vi "Begin.vi"(8 "error in":errorcluster) -> (0 "error out":errorcluster)   [LabVIEW 2019]
doc: "Called before other user functions, this VI is expected to open initial I/O refnums, load in file data, and do all program initialization. Notice that the <B>error out</B> terminal is simply used for data flow. Wiring it to other structures or subVIs ensures that this VI runs first."
uses:
  <vilib>/Rock Robotics/WPI/Camera/WPI_CameraImageSize.ctl
  <vilib>/Rock Robotics/WPI/Camera/WPI_CameraFrameRate.ctl
  <vilib>/Rock Robotics/WPI/Camera/WPI_CameraWhite Balance Values.ctl
  <vilib>/Rock Robotics/WPI/Camera/WPI_CameraExposure Values.ctl
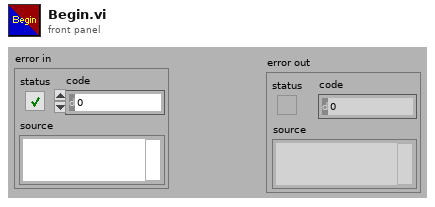
[diagram p1: front panel]
types:
  T1 = typedef "WPI_CameraExposure Values.ctl" = enum16{"Auto", "Flicker-free 50 Hz", "Flicker-free 60 Hz", "Hold current", "Custom"}
  T2 = typedef "WPI_CameraWhite Balance Values.ctl" = enum16{"Auto", "Fixed indoor", "Fixed outdoor 1", "Fixed outdoor 2", "Fixed fluorescent 1", "Fixed fluorescent 2", "Hold current", "Custom"}
  T3 = typedef "WPI_CameraFrameRate.ctl" = u32
  T4 = typedef "WPI_CameraImageSize.ctl" = enum16{"640x480", "320x240", "160x120", "Custom"}
  T5 = typedef "WPI_CameraDevRef.ctl" = cluster{"Camera Address":string, "CameraStatus":errorcluster}
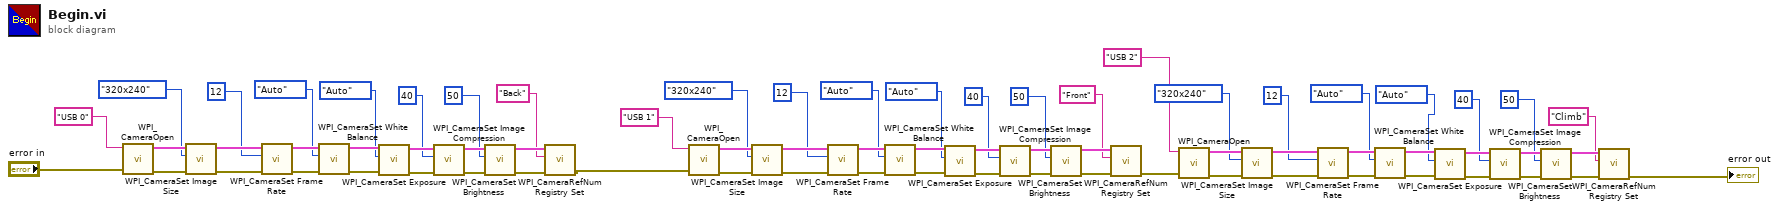
[diagram p0: block diagram]
diagram:
  n1 = call <vilib>:"WPI_CameraOpen.vi"("error in (no error)"="error in", "Camera Address"="USB 0") -> ("error out"=w68:errorcluster, "CameraDevRef"=w67:T5)  [unwired: 8 in]
  n2 = call <vilib>:"WPI_CameraSet Image Size.vi"("error in (no error)"=w68, "Image Size"=WPI_CameraImageSize."320x240", "CameraDevRef"=w67) -> ("error out"=w65:errorcluster, "CameraDevRef Out"=w64:T5)  [unwired: 7 in]
  n3 = call <vilib>:"WPI_CameraSet Frame Rate.vi"("error in (no error)"=w65, "Frame Rate (fps)"=T3 12, "CameraDevRef"=w64) -> ("error out"=w62:errorcluster, "CameraDevRef Out"=w61:T5)  [unwired: 7 in]
  n4 = call <vilib>:"WPI_CameraSet White Balance.vi"("error in (no error)"=w62, "White Balance"=WPI_CameraWhite_Balance_Values."Auto", "CameraDevRef"=w61) -> ("error out"=w59:errorcluster, "CameraDevRef Out"=w58:T5)  [unwired: 7 in]
  n5 = call <vilib>:"WPI_CameraSet Exposure.vi"("error in (no error)"=w59, "Exposure"=WPI_CameraExposure_Values."Auto", "CameraDevRef"=w58) -> ("error out"=w56:errorcluster, "CameraDevRef Out"=w55:T5)  [unwired: 7 in]
  n6 = call <vilib>:"WPI_CameraSet Image Compression.vi"("error in (no error)"=w56, "Compression"=40, "CameraDevRef"=w55) -> ("error out"=w53:errorcluster, "CameraDevRef Out"=w52:T5)  [unwired: 7 in]
  n7 = call <vilib>:"WPI_CameraSet Brightness.vi"("error in (no error)"=w53, "Brightness"=50, "CameraDevRef"=w52) -> ("error out"=w50:errorcluster, "CameraDevRef Out"=w49:T5)  [unwired: 7 in]
  n8 = call <vilib>:"WPI_CameraRefNum Registry Set.vi"("error in (no error)"=w50, "refnum name"="Back", "CameraDevRef"=w49) -> ("error out"=w25:errorcluster)  [unwired: 7 in, 1 out]
  n9 = call <vilib>:"WPI_CameraOpen.vi"("error in (no error)"=w25, "Camera Address"="USB 1") -> ("error out"=w46:errorcluster, "CameraDevRef"=w45:T5)  [unwired: 8 in]
  n10 = call <vilib>:"WPI_CameraSet Image Size.vi"("error in (no error)"=w46, "Image Size"=WPI_CameraImageSize."320x240", "CameraDevRef"=w45) -> ("error out"=w43:errorcluster, "CameraDevRef Out"=w42:T5)  [unwired: 7 in]
  n11 = call <vilib>:"WPI_CameraSet Frame Rate.vi"("error in (no error)"=w43, "Frame Rate (fps)"=T3 12, "CameraDevRef"=w42) -> ("error out"=w40:errorcluster, "CameraDevRef Out"=w39:T5)  [unwired: 7 in]
  n12 = call <vilib>:"WPI_CameraSet White Balance.vi"("error in (no error)"=w40, "White Balance"=WPI_CameraWhite_Balance_Values."Auto", "CameraDevRef"=w39) -> ("error out"=w37:errorcluster, "CameraDevRef Out"=w36:T5)  [unwired: 7 in]
  n13 = call <vilib>:"WPI_CameraSet Exposure.vi"("error in (no error)"=w37, "Exposure"=WPI_CameraExposure_Values."Auto", "CameraDevRef"=w36) -> ("error out"=w34:errorcluster, "CameraDevRef Out"=w33:T5)  [unwired: 7 in]
  n14 = call <vilib>:"WPI_CameraSet Image Compression.vi"("error in (no error)"=w34, "Compression"=40, "CameraDevRef"=w33) -> ("error out"=w31:errorcluster, "CameraDevRef Out"=w30:T5)  [unwired: 7 in]
  n15 = call <vilib>:"WPI_CameraSet Brightness.vi"("error in (no error)"=w31, "Brightness"=50, "CameraDevRef"=w30) -> ("error out"=w28:errorcluster, "CameraDevRef Out"=w27:T5)  [unwired: 7 in]
  n16 = call <vilib>:"WPI_CameraRefNum Registry Set.vi"("error in (no error)"=w28, "refnum name"="Front", "CameraDevRef"=w27) -> ("error out"=w5:errorcluster)  [unwired: 7 in, 1 out]
  n17 = call <vilib>:"WPI_CameraOpen.vi"("error in (no error)"=w5, "Camera Address"="USB 2") -> ("error out"=w24:errorcluster, "CameraDevRef"=w23:T5)  [unwired: 8 in]
  n18 = call <vilib>:"WPI_CameraSet Image Size.vi"("error in (no error)"=w24, "Image Size"=WPI_CameraImageSize."320x240", "CameraDevRef"=w23) -> ("error out"=w22:errorcluster, "CameraDevRef Out"=w21:T5)  [unwired: 7 in]
  n19 = call <vilib>:"WPI_CameraSet Frame Rate.vi"("error in (no error)"=w22, "Frame Rate (fps)"=T3 12, "CameraDevRef"=w21) -> ("error out"=w20:errorcluster, "CameraDevRef Out"=w19:T5)  [unwired: 7 in]
  n20 = call <vilib>:"WPI_CameraSet White Balance.vi"("error in (no error)"=w20, "White Balance"=WPI_CameraWhite_Balance_Values."Auto", "CameraDevRef"=w19) -> ("error out"=w18:errorcluster, "CameraDevRef Out"=w17:T5)  [unwired: 7 in]
  n21 = call <vilib>:"WPI_CameraSet Exposure.vi"("error in (no error)"=w18, "Exposure"=WPI_CameraExposure_Values."Auto", "CameraDevRef"=w17) -> ("error out"=w16:errorcluster, "CameraDevRef Out"=w15:T5)  [unwired: 7 in]
  n22 = call <vilib>:"WPI_CameraSet Image Compression.vi"("error in (no error)"=w16, "Compression"=40, "CameraDevRef"=w15) -> ("error out"=w14:errorcluster, "CameraDevRef Out"=w13:T5)  [unwired: 7 in]
  n23 = call <vilib>:"WPI_CameraSet Brightness.vi"("error in (no error)"=w14, "Brightness"=50, "CameraDevRef"=w13) -> ("error out"=w4:errorcluster, "CameraDevRef Out"=w3:T5)  [unwired: 7 in]
  n24 = call <vilib>:"WPI_CameraRefNum Registry Set.vi"("error in (no error)"=w4, "refnum name"="Climb", "CameraDevRef"=w3) -> ("error out"=→"error out":errorcluster)  [unwired: 7 in, 1 out]
